vi "stop.vi"(8 "error in (no error)":errorcluster, 10 "ElectrometerController int":refnum<class "ElectrometerController.lvclass">, 11 "SetDurationReading in":refnum<class "SetDurationReading.lvclass">) -> (0 "error out":errorcluster, 2 "ElectrometerController out":refnum<class "ElectrometerController.lvclass">, 3 "SetDurationReading out":refnum<class "SetDurationReading.lvclass">)   [LabVIEW 2016, in "SetDurationReading.lvclass"]
uses:
  SetDurationReading.lvclass
  ElectrometerController/ElectrometerController.lvclass
  internalState.ctl
  State.lvclass
  Electrometer.lvclass
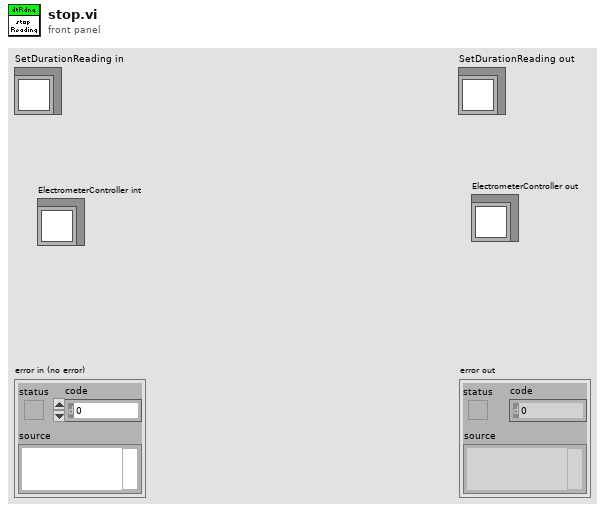
[diagram p1: front panel]
types:
  T1 = typedef "Electrometer.lvclass/internalState.ctl" = enum16{"Ready", "Configuring", "ManualReading", "UntilIntensityReading", "SetDurationReading"}
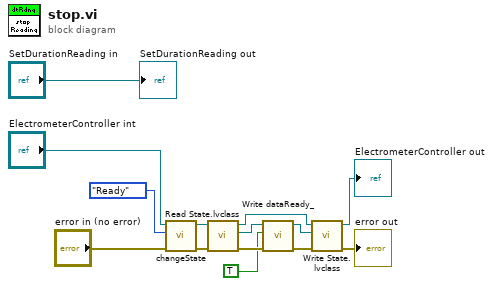
[diagram p0: block diagram]
diagram:
  n1 = call "changeState.vi"("error in (no error)"="error in (no error)", "State"=internalState."Ready" ("States"), "ElectrometerController in"="ElectrometerController int") -> ("error out"=w11:errorcluster, "ElectrometerController out"=w12:refnum<class "ElectrometerController.lvclass">)  [unwired: 7 in]
  n2 = call-dynamic "Read State.lvclass.vi"("error in (no error)"=w11, "ElectrometerController in"=w12) -> ("error out"=w9:errorcluster, "State.lvclass"=w10:refnum<class "State.lvclass">, "ElectrometerController out"=w6:refnum<class "ElectrometerController.lvclass">)  [unwired: 7 in]
  n3 = call-dynamic "Write dataReady_.vi"("error in (no error)"=w9, "dataReady?"=TRUE, "State in"=w10) -> ("error out"=w5:errorcluster, "State out"=w7:refnum<class "State.lvclass">)  [unwired: 7 in]
  n4 = call-dynamic "Write State.lvclass.vi"("error in (no error)"=w5, "State.lvclass"=w7, "ElectrometerController in"=w6) -> ("error out"=→"error out":errorcluster, "ElectrometerController out"=→"ElectrometerController out":refnum<class "ElectrometerController.lvclass">)  [unwired: 7 in]
  "SetDurationReading out" <- "SetDurationReading in"
